vi "Test JSON Parse.vi"() -> ()   [LabVIEW 2015]
doc: "Created IvanLis by LabVIEW Portal\nProfile: http://labviewportal.org/memberlist.php?mode=viewprofile&u=987\neMail: IvanLisanov@gMail.com\nTelegram: https://t.me/IvanLis"
uses:
  Telegram Library/TypeDef/Telegram State.ctl
  JSON Library/JSON Library.lvlib
  Telegram Library/Telegram Library.lvlib
panel:
  out "error out":errorcluster
  in  "Next":bool
  out "Message":variant
  out "Telegram State":T1
  out "Numeric":i32
  out "Message JSON":string
  in  "file (use dialog)":path=path "C:/Users/Ivan/Desktop/Telegram/Telegram-Clien_TDLib/log/log-83.json"
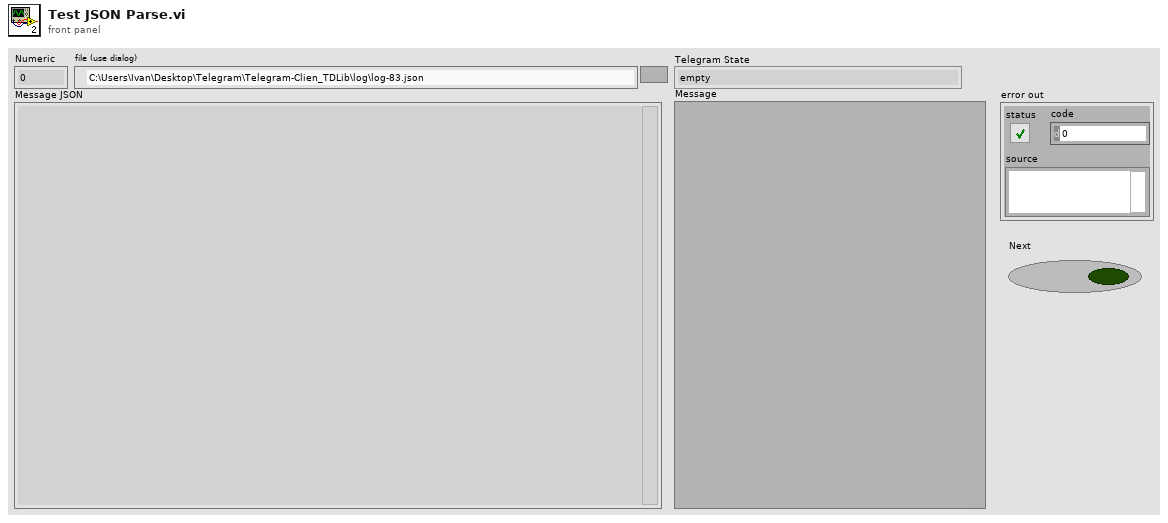
[diagram p1: front panel]
types:
  T1 = typedef "Telegram Library.lvlib/Telegram State.ctl" = enum16{"empty", "ok", "authorizationStateClosed", "authorizationStateWaitTdlibParameters", "authorizationStateWaitEncryptionKey", "authorizationStateWaitPhoneNumber", "authorizationStateWaitCode", "connectionStateWaitingForNetwork", "connectionStateConnectingToProxy", "connectionStateUpdating", "connectionStateConnecting", "connectionStateReady", "updateUser_user", "updateNewChat_chat", "updateNewMessage_Text", "updateChatLastMessage_message", "updateDeleteMessages", "updateChatPosition"}
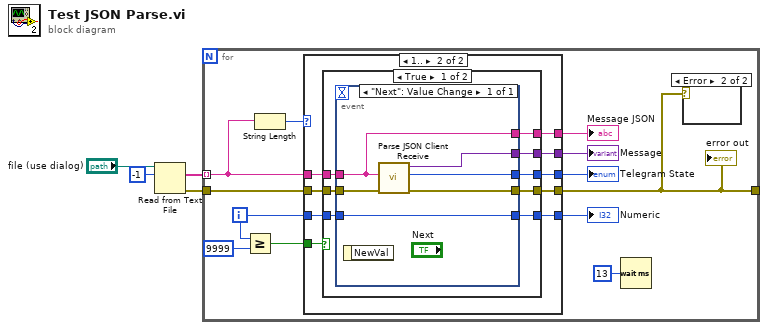
[diagram p0: block diagram]
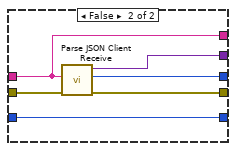
[diagram p3: hidden frame]
diagram:
  n1 = Read from Text File(file (use dialog)="file (use dialog)", count=-1) -> (text=w1:string[], error out=w2:errorcluster)  [unwired: 2 in, 2 out]
  n2 = for {
    tunnel: w1 -> [w8] mode=indexing
    tunnel: w2 -> [w16]
    tunnel: [w10] -> _
    i -> [w14]
    n3 = Greater Or Equal?(x=w14, y=9999) -> (x >= y?=w15:bool)
    n4 = String Length(string=w8) -> (length=w9:i32)
    n5 = case shown="1.." w9 {
      tunnel: w16 -> [w17 w26]
      tunnel: w8 -> [_ w25]
      tunnel: w15 -> [_ w24]
      tunnel: w14 -> [_ w23]
      tunnel: [_ w22] -> w12
      tunnel: [_ w21] -> w5
      tunnel: [_ w20] -> w6
      tunnel: [_ w19] -> w11
      tunnel: [w17 w18] -> w10
      frame ..0 {
      }
      frame 1.. {
        n6 = case shown="True" w24 {
          tunnel: w26 -> [w34 w43]
          tunnel: w25 -> [w33 w42]
          tunnel: w23 -> [w32 w44]
          tunnel: [w31 w41] -> w18
          tunnel: [w30 w42] -> w22
          tunnel: [w29 w46] -> w21
          tunnel: [w28 w45] -> w20
          tunnel: [w27 w44] -> w19
          frame True {
            n7 = event shown="[0] \"Next\": Value Change" {
              selector: _ -> [_]
              dyn-events: _ -> [_]
              timeout: _ -> [_]
              tunnel: w34 -> [w37]
              tunnel: w33 -> [w36]
              tunnel: [w35] -> w31
              tunnel: w32 -> [w38]
              tunnel: [w36] -> w30
              tunnel: [w40] -> w29
              tunnel: [w39] -> w28
              tunnel: [w38] -> w27
              event "Next": Value Change {
                n8 = event-data() -> ()  [unwired: 1 in, 1 out]
                n9 = call "Parse JSON Client Receive.vi"("error in (no error)"=w37, "JSON (UTF-8) String"=w36) -> ("error out"=w35:errorcluster, "Telegram State"=w39:T1, "Message"=w40:variant)  [unwired: 7 in]
              }
            }
          }
          frame False {
            n10 = call "Parse JSON Client Receive.vi"("error in (no error)"=w43, "JSON (UTF-8) String"=w42) -> ("error out"=w41:errorcluster, "Telegram State"=w45:T1, "Message"=w46:variant)  [unwired: 7 in]
          }
        }
      }
    }
    "error out" <- w10
    "Message JSON" <- w12
    "Numeric" <- w11
    "Telegram State" <- w6
    "Message" <- w5
    n11 = Wait (ms)(milliseconds to wait=u32 13) -> ()  [unwired: 1 out]
    n12 = case shown="Error" w10 {
      frame No Error {
      }
      frame Error {
      }
    }
  }
